vi "digest test.vi"() -> ()   [LabVIEW 2016]
uses:
  libretls/crypto digest/lvlibcrypto digest.lvclass
panel:
  out "digest":string
  out "error out":errorcluster
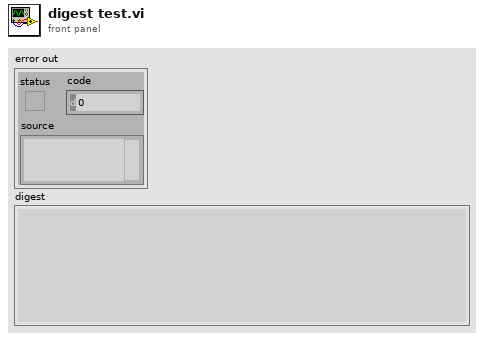
[diagram p1: front panel]
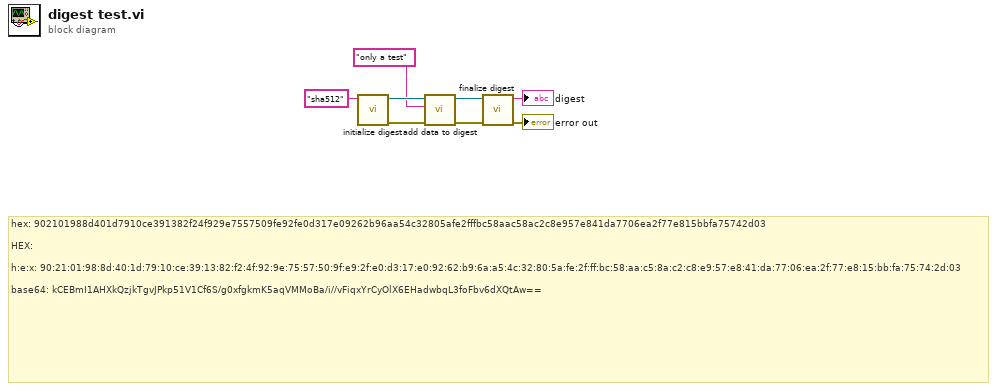
[diagram p0: block diagram]
diagram:
  # "hex: 902101988d401d7910ce391382f24f929e7557509fe92fe0d317e09262b96aa54c32805afe2fffbc58aac58ac2c8e957e841da7706ea2f77e815bbfa75742d03\n\nHEX: \n\nh:e:x: 90:21:01:98:8d:40:1d:79:10:ce:39:13:82:f2:4f:92:9e:75:57:50:9f:e9:2f:e0:d3:17:e0:92:62:b9:6a:a5:4c:32:80:5a:fe:2f:ff:bc:58:aa:c5:8a:c2:c8:e9:57:e8:41:da:77:06:ea:2f:77:e8:15:bb:fa:75:74:2d:03\n\nbase64: kCEBmI1AHXkQzjkTgvJPkp51V1Cf6S/g0xfgkmK5aqVMMoBa/i//vFiqxYrCyOlX6EHadwbqL3foFbv6dXQtAw=="
  n1 = call "initialize digest.vi"("digest name"="sha512") -> ("error out"=w7:errorcluster, "lvlibcrypto digest out"=w8:refnum<class "lvlibcrypto digest.lvclass">)  [unwired: 9 in]
  n2 = call "add data to digest.vi"("error in"=w7, "data to add"="only a test", "lvlibcrypto digest in"=w8) -> ("error out"=w5:errorcluster, "lvlibcrypto digest out"=w6:refnum<class "lvlibcrypto digest.lvclass">)  [unwired: 7 in]
  n3 = call "finalize digest.vi"("error in"=w5, "lvlibcrypto digest in"=w6) -> ("error out"=→"error out":errorcluster, "digest"=→"digest":string)  [unwired: 8 in]
